vi "Teleop.vi"(10 "Match Info":T1={"Autonomous Elapsed Seconds"=0.0, "TeleOp Elapsed Seconds"=0.0, "Disabled Elapsed Seconds"=0.0, "Visited Autonomous"=FALSE, "Visited TeleOp"=FALSE, "Visited Disabled"=FALSE, "Autonomous Settings"={"Autonomous Style"=enum."Independent", "VI Refnum"=refnum}}, 11 "Call Context":T2) -> ()   [LabVIEW 2017]
doc: "This VI is called for each TeleOp packet received from the DS where the robot is not disabled. It is often used to read from the joysticks and update I/O or to update setpoints for timed control loops. It should complete and return within 20 milliseconds or it may miss DS packets."
uses:
  <vilib>/Rock Robotics/WPI/DriverStation/WPI_DriverStationDerivedRobotMode.ctl
  <vilib>/Rock Robotics/WPI/DriverStation/WPI_DriverStationMatch Info.ctl
  TypeDef/ENUM_WC_Drive_DriveMode.ctl
  _SHARE ALL/RoboRio Share All/Systems Share All/Joystick/Global_Joystick Write_Data.vi
  Globals/Global_CMD_Gear.vi
  Globals/Global_CMD_Drive.vi
  _SHARE ALL/RoboRio Share All/Systems Share All/Joystick/Joystick.lvlib
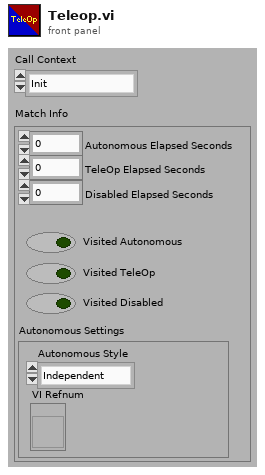
[diagram p1: front panel]
types:
  T1 = typedef "WPI_DriverStationMatch Info.ctl" = cluster{"Autonomous Elapsed Seconds":dbl, "TeleOp Elapsed Seconds":dbl, "Disabled Elapsed Seconds":dbl, "Visited Autonomous":bool, "Visited TeleOp":bool, "Visited Disabled":bool, "Autonomous Settings":cluster{"Autonomous Style":enum16{"Iterative", "Independent"}, "VI Refnum":refnum<vi>}}
  T2 = typedef "WPI_DriverStationDerivedRobotMode.ctl" = enum16{"Init", "Execute", "Stop"}
  T3 = typedef "ENUM_WC_Drive_DriveMode.ctl" = enum16{"Motion Profile", "CrossLineAuto", "VBus", "Stop"}
  T4 = typedef "CLUSTER_CMD_WC_Drive.ctl" = cluster{"Drive_Mode":T3, "VBus":T5, "Profile":T7}
  T5 = typedef "CLUSTER_Drive_ACT Loop_VBus Data.ctl" = cluster{"Drive":T6, "Turbo":bool}
  T6 = typedef "CLUSTER_X and Y.ctl" = cluster{"Steer":dbl, "Throtle":dbl}
  T7 = typedef "CLUSTER_Drive_ACT Loop_Profile Data.ctl" = cluster{"Start":bool}
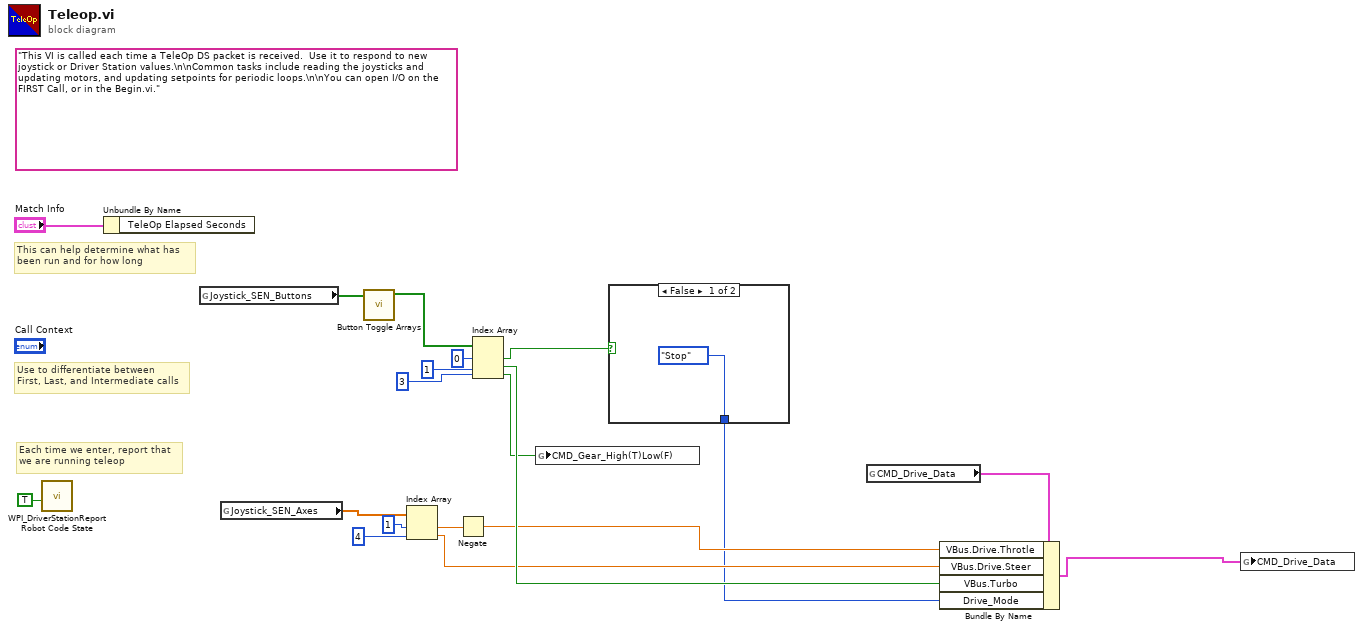
[diagram p0: block diagram]
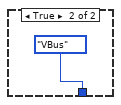
[diagram p2: hidden frame]
diagram:
  (unwired) "This VI is called each time a TeleOp DS packet is received.  Use it to respond to new joystick or Driver Station values.\n\nCommon tasks include reading the joysticks and updating motors, and updating setpoints for periodic loops.\n\nYou can open I/O on the FIRST Call, or in the Begin.vi."
  # "Each time we enter, report that\nwe are running teleop"
  # "Use to differentiate between\nFirst, Last, and Intermediate calls"
  # "This can help determine what has\nbeen run and for how long"
  n1 = call <vilib>:"WPI_DriverStationReport Robot Code State.vi"("TeleOp"=TRUE ("Autonomous")) -> ()  [unwired: 10 in, 1 out]
  n2 = Unbundle By Name("Match Info") -> ()  [unwired: 1 out]
  n3 = global read "Global_Joystick Write_Data.vi" "Joystick_SEN_Buttons"() -> (w5:bool[])
  n4 = global read "Global_Joystick Write_Data.vi" "Joystick_SEN_Axes"() -> (w15:dbl[])
  n5 = call "Button Toggle Arrays.vi"("Joystick_SEN_Buttons"=w5) -> ("Toggle Outputs Out"=w4:bool[])  [unwired: 8 in, 2 out]
  n6 = Index Array(array=w15, index #1=1 ("index"), index #2=4 ("index")) -> (element #1=w9:dbl, element #2=w11:dbl)
  n7 = Negate(x=w9) -> (-x=w8:dbl)
  n8 = Index Array(array=w4, index #1=0 ("index"), index #2=1 ("index"), index #3=3 ("index")) -> (element #1=w17:bool, element #2=w13:bool, element #3=w2:bool)
  n9 = global write "Global_CMD_Gear.vi" "CMD_Gear_High(T)Low(F)"(w2) -> ()
  n10 = case shown="False" w17 {
    tunnel: [ENUM_WC_Drive_DriveMode."Stop" ("Drive_Mode") ENUM_WC_Drive_DriveMode."VBus" ("Drive_Mode")] -> w1
    frame False {
    }
    frame True {
    }
  }
  n11 = global read "Global_CMD_Drive.vi" "CMD_Drive_Data"() -> (w7:T4)
  n12 = Bundle By Name(cluster=w7, "VBus.Drive.Throtle"=w8, "VBus.Drive.Steer"=w11, "VBus.Turbo"=w13, "Drive_Mode"=w1) -> (w6:T4)
  n13 = global write "Global_CMD_Drive.vi" "CMD_Drive_Data"(w6) -> ()
